vi "NewRobotTurningAroundBallDev.vi"(7 "firstCall?":bool, 8 "Target":dbl[](array[numeric]), 9 "KickToSkill in":refnum<class "KickToSkill.lvclass">, 10 "Game":refnum<class "Game.lvclass">, 11 "Robot in":refnum<class "Robot.lvclass">) -> (2 "KickToSkill out":refnum<class "KickToSkill.lvclass">, 3 "Robot out":refnum<class "Robot.lvclass">)   [LabVIEW 2021, in "KickToSkill.lvclass"]
uses:
  KickToSkill.lvclass
  Game_class/Game.lvclass
  Robot_class/Robot.lvclass
  robotTurningAroundBallStates.ctl
  Object_class/Object.lvclass/Object.ctl
  Game_class/Game.lvclass/Game.ctl
  Robot_class/Robot.lvclass/Robot.ctl
  <vilib>/Analysis/baseanly.llb/Unit Vector (DBL).vi
  <vilib>/Analysis/coordinate.llb/2D Cartesian Coordinate Rotation (Scalar).vi
  Robot_class/Read dest_x.vi
  Robot_class/Read dest_y.vi
  Robot_class/Read dest_orientation.vi
  Robot_class/Read kick_x.vi
  Robot_class/Read orientation.vi
  Game_class/Read BallRef.vi
  Object_class/Read position(x,y).vi
  Object_class/Read x.vi
  Robot_class/Write dest_orientation.vi
  Robot_class/Write dest_x.vi
  Robot_class/Write dest_y.vi
  Robot_class/Write kick_x.vi
  Robot_class/Write dribble.vi
  Ball_class/Ball.lvclass
  <vilib>/Analysis/NI_AALPro.lvlib
  <vilib>/Analysis/NI_AALBase.lvlib
panel:
  in  "Raio":dbl=200.0
  out "error out":errorcluster
  in  "error in (no error)":errorcluster
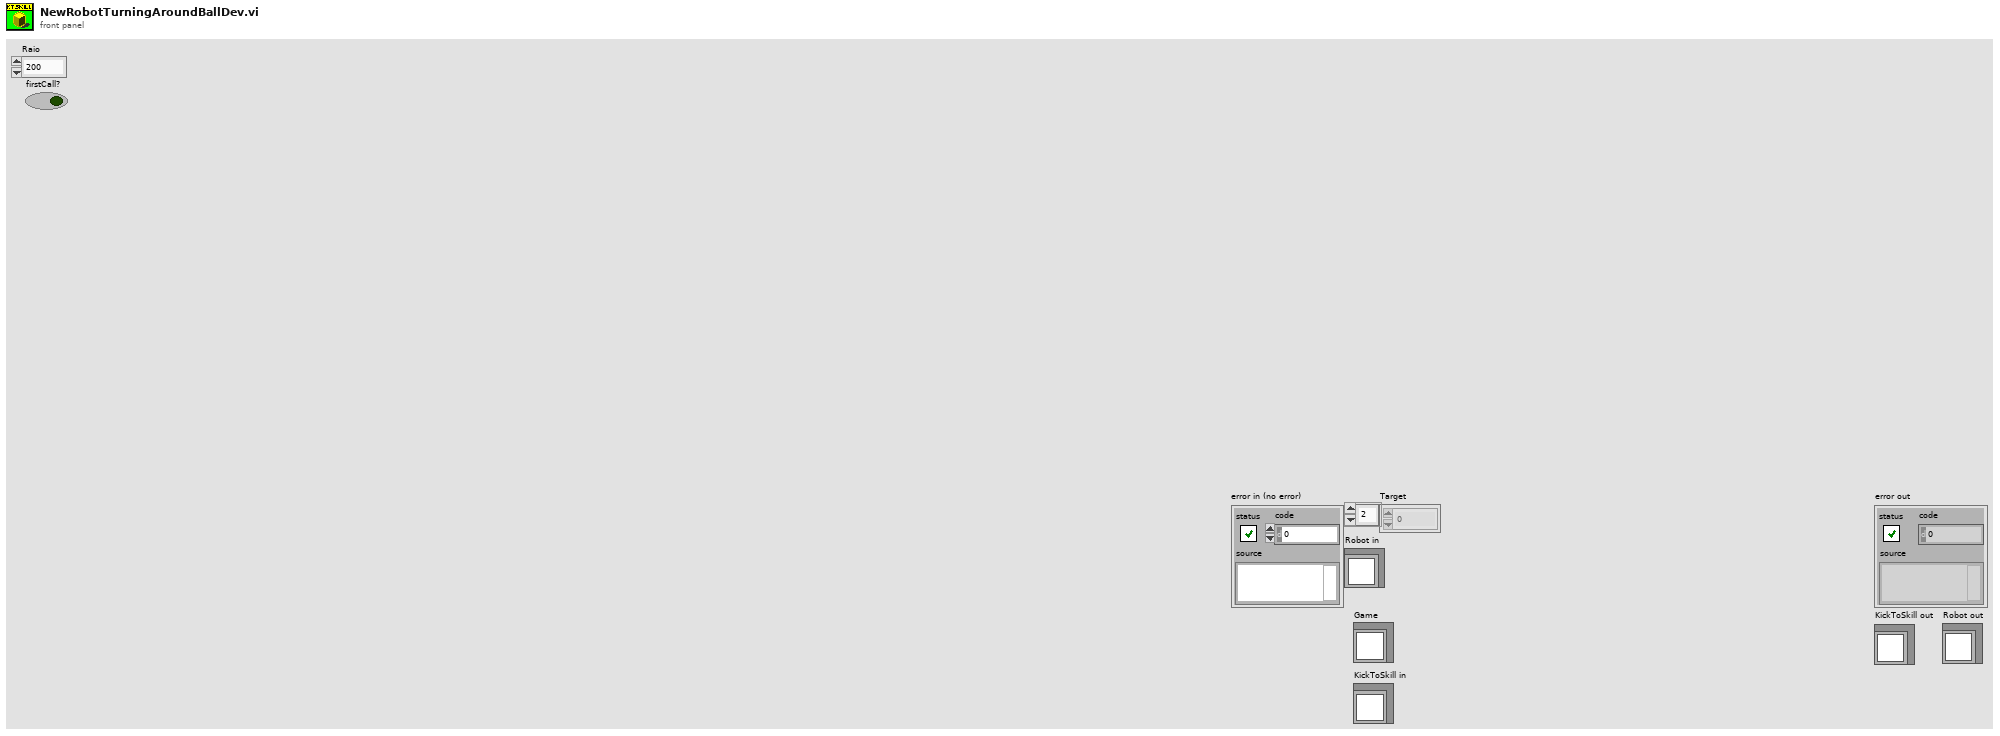
[diagram p1: front panel]
types:
  T1 = typedef "KickToSkill.lvclass/robotTurningAroundBallStates.ctl" = enum16{"go straight to the target", "go to point A", "circulating the ball", "take distance", "lining up", "shoot"}
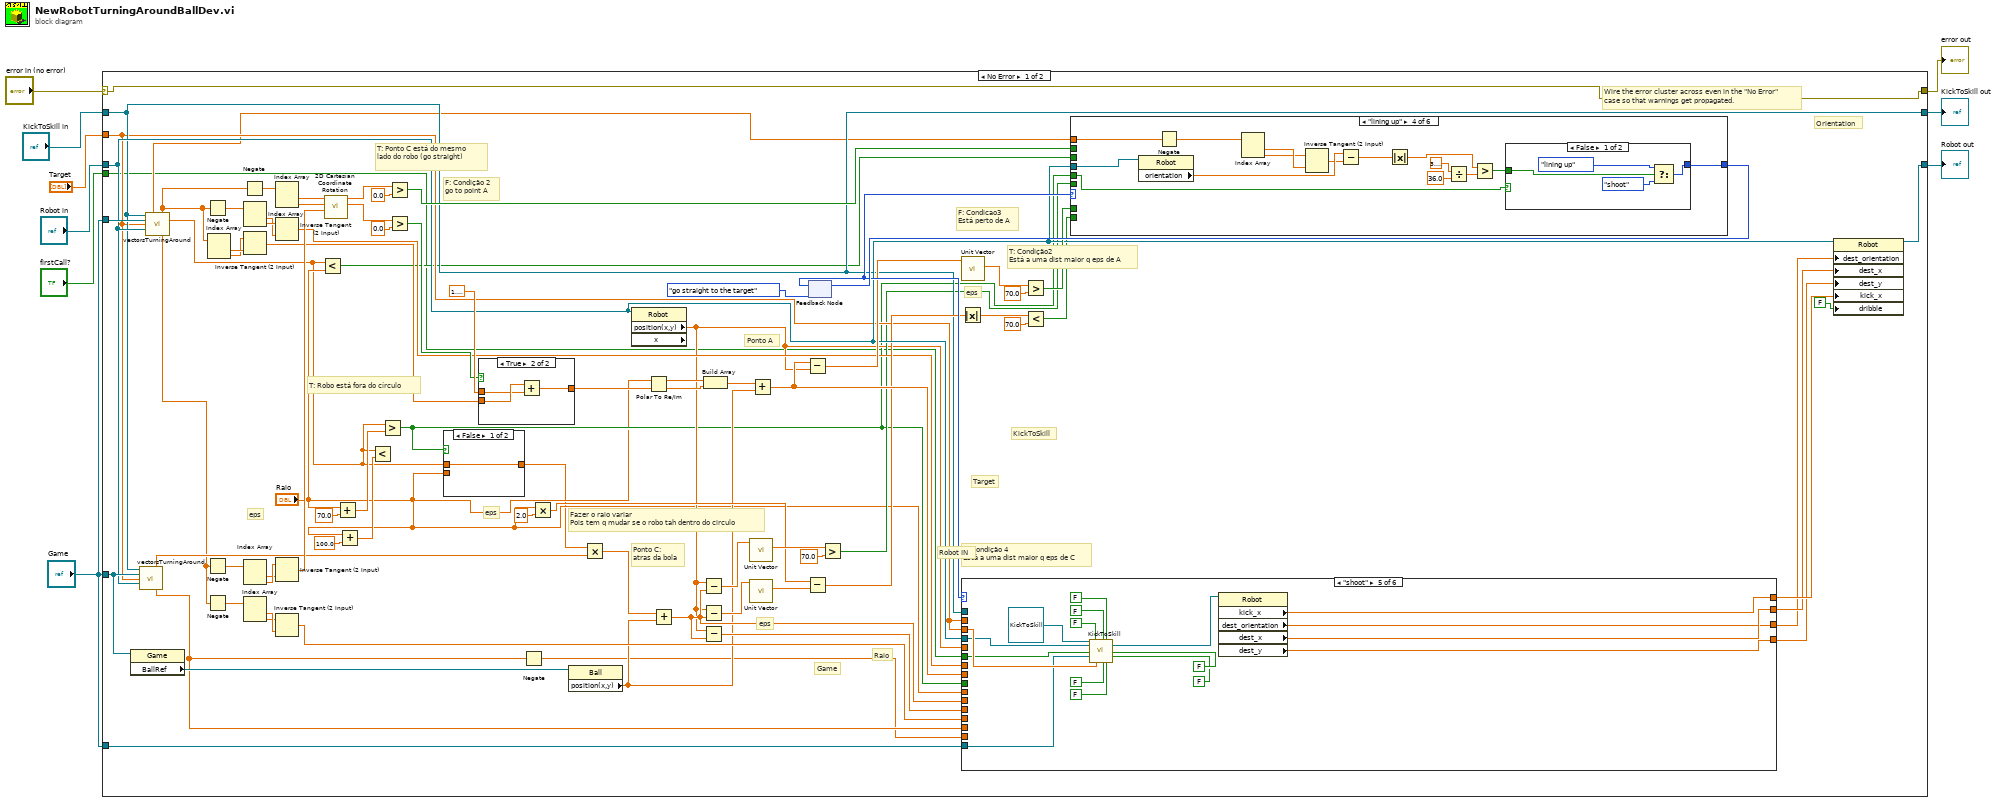
[diagram p0: block diagram]
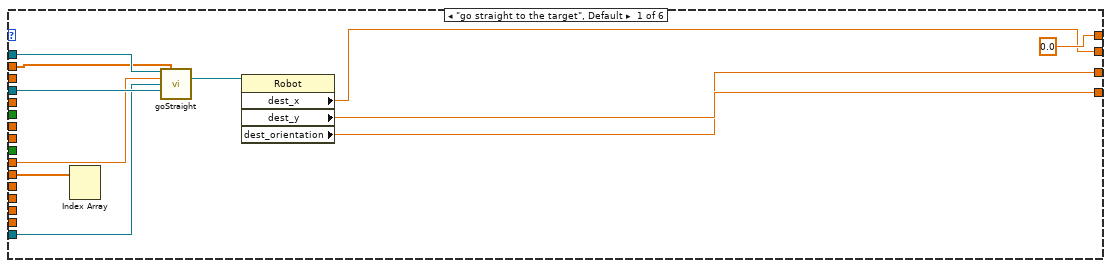
[diagram p3: hidden frame]
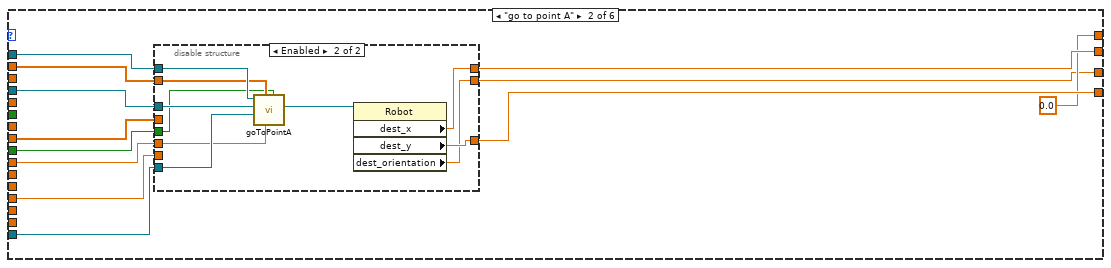
[diagram p4: hidden frame]
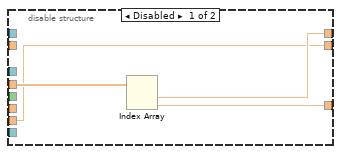
[diagram p5: hidden frame]
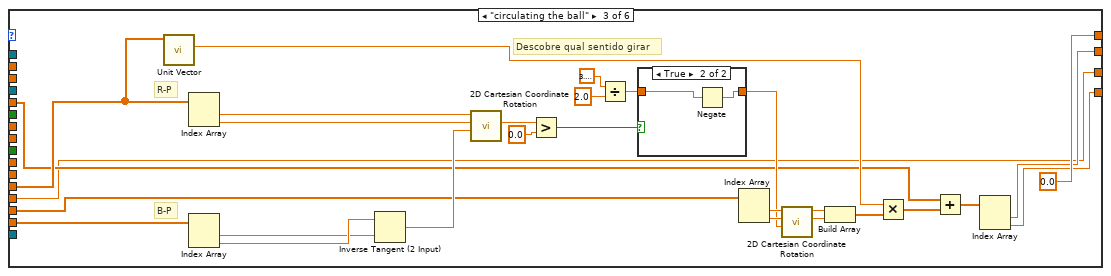
[diagram p6: hidden frame]
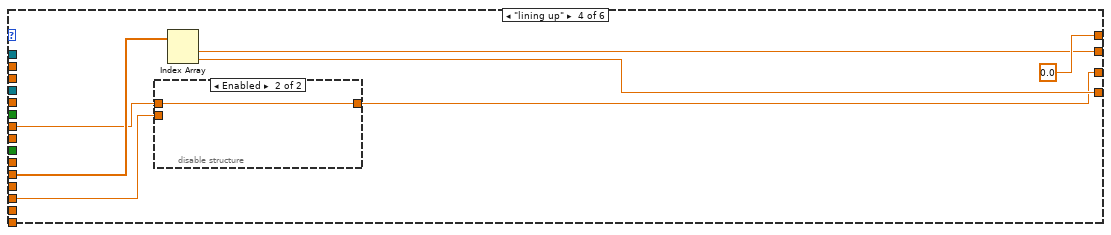
[diagram p8: hidden frame]
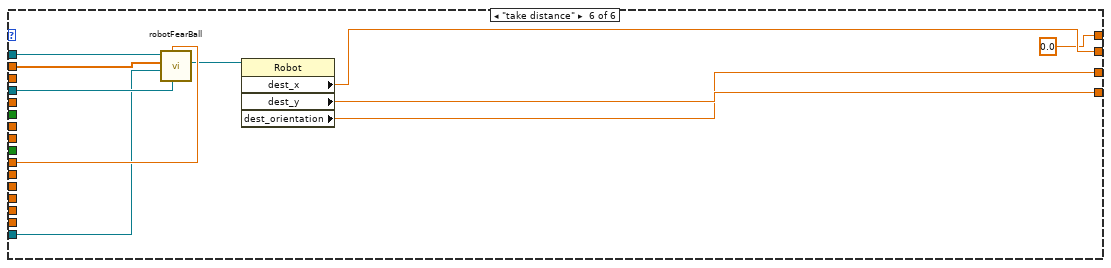
[diagram p10: hidden frame]
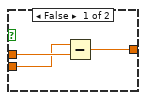
[diagram p11: hidden frame]
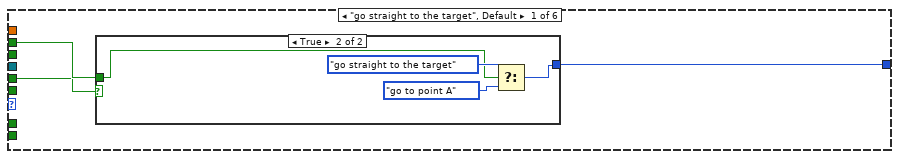
[diagram p12: hidden frame]
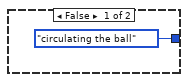
[diagram p13: hidden frame]
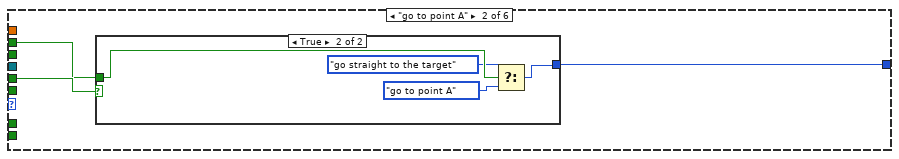
[diagram p14: hidden frame]
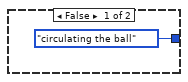
[diagram p15: hidden frame]
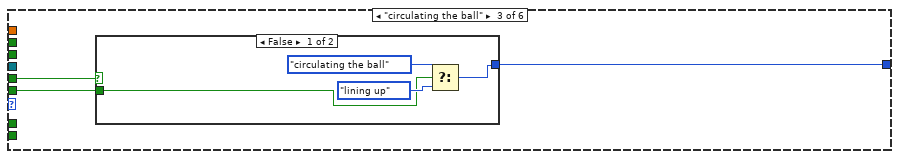
[diagram p16: hidden frame]
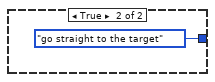
[diagram p17: hidden frame]
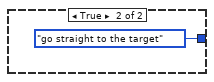
[diagram p18: hidden frame]
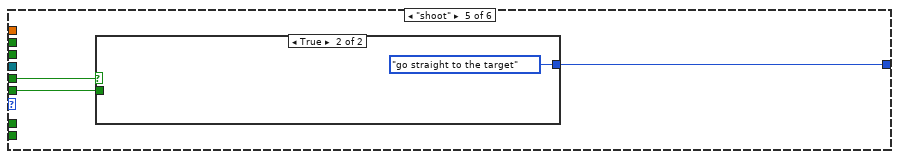
[diagram p19: hidden frame]
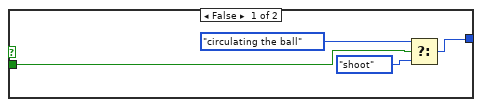
[diagram p20: hidden frame]
diagram:
  n1 = case shown="No Error" "error in (no error)" {
    selector: "error in (no error)" -> [w93 w268]
    tunnel: [w93 w268] -> w8
    tunnel: [w29 w267] -> w6
    tunnel: "KickToSkill in" -> [w29 w267]
    tunnel: "Robot in" -> [w45 w266]
    tunnel: [w92 w266] -> w4
    tunnel: "Target" -> [w28 _]
    tunnel: "Game" -> [w89 _]
    tunnel: "Game" -> [w46 _]
    tunnel: "Game" -> [w50 _]
    tunnel: "firstCall?" -> [w10 _]
    frame No Error {
      # "Fazer o raio variar\nPois tem q mudar se o robo tah dentro do circulo"
      # "Orientation"
      # "Raio"
      # "Robot IN"
      # "Game"
      # "KickToSkill"
      # "Target"
      # "eps"
      # "T: Condição 4\nEstá a uma dist maior q eps de C"
      # "F: Condicao3\nEstá perto de A"
      # "eps"
      # "Ponto C:\natras da bola"
      # "eps"
      # "eps"
      # "F: Condição 2\ngo to point A"
      # "T: Condição2\nEstá a uma dist maior q eps de A"
      # "Ponto A"
      # "T: Robo está fora do círculo"
      # "T: Ponto C está do mesmo lado do robo (go straight)"
      # "Wire the error cluster across even in the \"No Error\"\ncase so that warnings get propagated."
      n2 = property class="Game"(reference=w46) -> ("BallRef"=w68:refnum<class "Ball.lvclass">)  [unwired: 1 in, 2 out]
      n3 = call "vectorsTurningAround.vi"("KickToSkill in"=w29, "Game"=w46, "Target"=w28, "Robot in"=w45) -> ("B-T"=w69:dbl[], "R-B"=w31:dbl[])  [unwired: 4 in, 6 out]
      n4 = call "vectorsTurningAround.vi"("KickToSkill in"=w29, "Game"=w89, "Target"=w28, "Robot in"=w45) -> ("R-T"=w16:dbl[], "B-T"=w22:dbl[], "R-B norm"=w11:dbl, "R-B"=w34:dbl[])  [unwired: 4 in, 4 out]
      n5 = Negate(x=w22) -> (-x=w25:dbl[])
      n6 = Negate(x=w34) -> (-x=w33:dbl[])
      n7 = Negate(x=w34) -> (-x=w44:dbl[])
      n8 = Index Array(array=w22) -> (element #1=w80:dbl, element #2=w79:dbl)  [unwired: 2 in]
      n9 = Negate(x=w22) -> (-x=w78:dbl[])
      n10 = Index Array(array=w25) -> (element #1=w23:dbl, element #2=w24:dbl)  [unwired: 2 in]
      n11 = Inverse Tangent (2 Input)(1:w80, 2:w79) -> (0:w77:dbl)
      n12 = Index Array(array=w33) -> (element #1=w83:dbl, element #2=w84:dbl)  [unwired: 2 in]
      n13 = Index Array(array=w44) -> (element #1=w57:dbl, element #2=w56:dbl)  [unwired: 2 in]
      n14 = Index Array(array=w78) -> (element #1=w85:dbl, element #2=w86:dbl)  [unwired: 2 in]
      n15 = Inverse Tangent (2 Input)(1:w23, 2:w24) -> (0:w21:dbl)
      n16 = Inverse Tangent (2 Input)(1:w83, 2:w84) -> (0:w82:dbl)
      n17 = Inverse Tangent (2 Input)(1:w57, 2:w56) -> (0:w48:dbl)
      n18 = Less?(x=w11, y="Raio") -> (x < y?=w20:bool)
      n19 = call-poly <vilib>:"2D Cartesian Coordinate Rotation.vi"("theta"=w82, "y"=w86, "x"=w85) -> ("y out"=w75:dbl, "x out"=w87:dbl)  [unwired: 6 in, 1 out]
      n20 = Add(x="Raio", y=70.0) -> (x+y=w18:dbl)
      n21 = Add(x="Raio", y=100.0) -> (x+y=w26:dbl)
      n22 = Less?(x=w11, y=w26) -> ()  [unwired: 1 out]
      n23 = Greater?(x=w11, y=w18) -> (0:w14:bool)
      n24 = Greater?(x=w87, y=0.0) -> (0:w81:bool)
      n25 = Greater?(x=w75, y=0.0) -> (0:w73:bool)
      n26 = case shown="False" w14 {
        tunnel: "Raio" -> [_ w95]
        tunnel: [w94 w95] -> w12
        tunnel: w11 -> [w94 _]
        frame False {
        }
        frame True {
        }
      }
      n27 = case shown="True" w73 {
        tunnel: w77 -> [w201 w205]
        tunnel: 1.5707963267948966 -> [w202 w204]
        tunnel: [w200 w203] -> w63
        frame False {
          n28 = Subtract(x=w201, y=w202) -> (x-y=w200:dbl)
        }
        frame True {
          n29 = Add(x=w205, y=w204) -> (x+y=w203:dbl)
        }
      }
      n30 = Negate(x=w31) -> (-x=w30:dbl[])
      n31 = Multiply(x="Raio", y=2.0) -> (x*y=w39:dbl)
      n32 = property class="Ball"(reference=w68) -> ("position(x,y)"=w32:dbl[])  [unwired: 1 in, 2 out]
      n33 = Multiply(x=w12, y=w69) -> (x*y=w67:dbl[])
      n34 = property class="Robot" props=["position(x,y)", "x"](reference=w45) -> ("position(x,y)"=w15:dbl[])  [unwired: 1 in, 3 out]
      n35 = Polar To Re/Im(2:w63, 3:"Raio") -> (0:w61:dbl, 1:w62:dbl)
      n36 = Add(x=w67, y=w32) -> (x+y=w43:dbl[])
      n37 = Subtract(x=w15, y=w43) -> (x-y=w58:dbl[])
      n38 = Subtract(x=w15, y=w43) -> (x-y=w42:dbl[])
      n39 = Subtract(x=w15, y=w43) -> (x-y=w51:dbl[])
      n40 = Build Array(w62, w61) -> (w60:dbl[])
      n41 = call-poly <vilib>:"Unit Vector.vi"("Input Vector"=w58) -> ("norm"=w65:dbl)  [unwired: 8 in, 2 out]
      n42 = call-poly <vilib>:"Unit Vector.vi"("Input Vector"=w42) -> ("norm"=w41:dbl)  [unwired: 8 in, 2 out]
      n43 = Add(x=w60, y=w32) -> (x+y=w59:dbl[])
      n44 = Subtract(x=w59, y=w15) -> (x-y=w47:dbl[])
      n45 = Subtract(x=w39, y=w41) -> (x-y=w38:dbl)
      n46 = feedback #1(robotTurningAroundBallStates."go straight to the target") -> (w64:T1)
      n47 = Greater?(x=w65, y=70.0) -> (0:w17:bool)
      n48 = Absolute Value(x=w38) -> (abs(x)=w37:dbl)
      n49 = call-poly <vilib>:"Unit Vector.vi"("Input Vector"=w47) -> ("norm"=w71:dbl)  [unwired: 8 in, 2 out]
      n50 = case shown="\"shoot\"" w64 {
        tunnel: w59 -> [_ w118 _ _ _ _]
        tunnel: [0.0 ("kick_x") 0.0 ("kick_x") 0.0 ("kick_x") 0.0 ("kick_x") w173 0.0 ("kick_x")] -> w54
        tunnel: w43 -> [w105 _ _ w169 _ _]
        tunnel: [w99 w117 w135 w168 w177 w193] -> w53
        tunnel: [w98 w116 w134 w167 w176 w192] -> w52
        tunnel: w30 -> [_ _ w143 _ _ _]
        tunnel: w51 -> [_ _ w141 _ _ _]
        tunnel: w31 -> [_ _ w142 _ _ _]
        tunnel: w15 -> [_ _ w138 _ _ _]
        tunnel: w28 -> [_ _ _ _ w181 _]
        tunnel: w45 -> [w103 w114 _ _ w180 w196]
        tunnel: w50 -> [w96 w113 _ _ w179 w195]
        tunnel: w48 -> [_ w108 w133 w166 _ _]
        tunnel: [w97 w109 w133 w165 w175 w190] -> w49
        tunnel: w29 -> [w104 w115 _ _ _ w197]
        tunnel: "Raio" -> [w102 w112 _ _ _ w198]
        tunnel: w28 -> [w101 w111 _ _ _ w199]
        tunnel: w21 -> [_ _ _ w164 _ _]
        tunnel: w14 -> [_ w107 _ _ _ _]
        tunnel: w10 -> [_ _ _ _ w174 _]
        frame "go straight to the target", Default {
          n51 = Index Array(array=w105) -> ()  [unwired: 2 in, 2 out]
          n52 = call "goStraight.vi"("KickToSkill in"=w104, "Target"=w101, "Raio"=w102, "Game"=w96, "Robot in"=w103) -> ("Robot out"=w100:refnum<class "Robot.lvclass">)  [unwired: 8 in, 2 out]
          n53 = property class="Robot"(reference=w100) -> ("dest_x"=w99:dbl, "dest_y"=w98:dbl, "dest_orientation"=w97:dbl)  [unwired: 1 in, 2 out]
        }
        frame "go to point A" {
          n54 = disable-structure shown="Enabled" {
            disable-tunnel: w118 -> [w122 _]
            disable-tunnel: [w121 w126] -> w117
            disable-tunnel: [w120 w125] -> w116
            disable-tunnel: w115 -> [_ w132]
            disable-tunnel: w114 -> [_ w131]
            disable-tunnel: w113 -> [_ w130]
            disable-tunnel: w112 -> [_ w129]
            disable-tunnel: w111 -> [_ w128]
            disable-tunnel: [w119 w124] -> w109
            disable-tunnel: w108 -> [w119 _]
            disable-tunnel: w107 -> [_ w123]
            frame Disabled {
              n55 = Index Array(array=w122) -> (element #1=w121:dbl, element #2=w120:dbl)  [unwired: 2 in]
            }
            frame Enabled {
              n56 = call "goToPointA.vi"("Fora do circulo"=w123, "Raio"=w129, "Target"=w128, "Game"=w130, "Robot in"=w131, "KickToSkill in"=w132) -> ("Robot out"=w127:refnum<class "Robot.lvclass">)  [unwired: 3 in, 2 out]
              n57 = property class="Robot"(reference=w127) -> ("dest_x"=w126:dbl, "dest_y"=w125:dbl, "dest_orientation"=w124:dbl)  [unwired: 1 in, 2 out]
            }
          }
        }
        frame "circulating the ball" {
          # "B-P"
          # "R-P"
          # "Descobre qual sentido girar"
          n58 = call-poly <vilib>:"Unit Vector.vi"("Input Vector"=w141) -> ("norm"=w140:dbl)  [unwired: 8 in, 2 out]
          n59 = Index Array(array=w141) -> (element #1=w151:dbl, element #2=w150:dbl)  [unwired: 2 in]
          n60 = Index Array(array=w143) -> (element #1=w144:dbl, element #2=w145:dbl)  [unwired: 2 in]
          n61 = Inverse Tangent (2 Input)(1:w144, 2:w145) -> (0:w149:dbl)
          n62 = call-poly <vilib>:"2D Cartesian Coordinate Rotation.vi"("theta"=w149, "y"=w150, "x"=w151) -> ("y out"=w148:dbl)  [unwired: 6 in, 2 out]
          n63 = Greater?(x=w148, y=0.0) -> (0:w146:bool)
          n64 = Divide(x=3.141592653589793, y=2.0) -> (x/y=w153:dbl)
          n65 = case shown="True" w146 {
            tunnel: w153 -> [w161 w163]
            tunnel: [w161 w162] -> w152
            frame False {
            }
            frame True {
              n66 = Negate(x=w163) -> (-x=w162:dbl)
            }
          }
          n67 = Index Array(array=w142) -> (element #1=w159:dbl, element #2=w158:dbl)  [unwired: 2 in]
          n68 = call-poly <vilib>:"2D Cartesian Coordinate Rotation.vi"("theta"=w152, "y"=w158, "x"=w159) -> ("y out"=w156:dbl, "x out"=w157:dbl)  [unwired: 6 in, 1 out]
          n69 = Build Array(w157, w156) -> (w139:dbl[])
          n70 = Multiply(x=w140, y=w139) -> (x*y=w137:dbl[])
          n71 = Add(x=w138, y=w137) -> (x+y=w136:dbl[])
          n72 = Index Array(array=w136) -> (element #1=w135:dbl, element #2=w134:dbl)  [unwired: 2 in]
        }
        frame "lining up" {
          n73 = disable-structure shown="Enabled" {
            disable-tunnel: w166 -> [w171 _]
            disable-tunnel: [w171 w172] -> w165
            disable-tunnel: w164 -> [_ w172]
            frame Disabled {
            }
            frame Enabled {
            }
          }
          n74 = Index Array(array=w169) -> (element #1=w168:dbl, element #2=w167:dbl)  [unwired: 2 in]
        }
        frame "shoot" {
          n75 = call "KickToSkill.vi"("KickToSkill in"=refnum<class "KickToSkill.lvclass"> refnum, "Robot"=w180, "firstCall?"=w174, "Game"=w179, "use criteria?"=FALSE, "Target"=w181, "chipKick ?"=FALSE, "KickForce 0?"=FALSE, "WeakKick"=FALSE, "ForceInGame"=FALSE, "IgnorePosEst"=FALSE, "pass?"=FALSE) -> ("Robot out"=w183:refnum<class "Robot.lvclass">)  [unwired: 4 in, 3 out]
          n76 = property class="Robot"(reference=w183) -> ("kick_x"=w173:dbl, "dest_orientation"=w175:dbl, "dest_x"=w177:dbl, "dest_y"=w176:dbl)  [unwired: 1 in, 2 out]
        }
        frame "take distance" {
          n77 = call "robotFearBall.vi"("Robot in"=w196, "Raio"=w198, "Game"=w195, "Target"=w199, "KickToSkill in"=w197) -> ("Robot out"=w194:refnum<class "Robot.lvclass">)  [unwired: 4 in, 2 out]
          n78 = property class="Robot"(reference=w194) -> ("dest_x"=w193:dbl, "dest_y"=w192:dbl, "dest_orientation"=w190:dbl)  [unwired: 1 in, 2 out]
        }
      }
      n79 = Greater?(x=w71, y=70.0) -> (0:w70:bool)
      n80 = Less?(x=w37, y=70.0) -> (x < y?=w35:bool)
      n81 = case shown="\"lining up\"" w64 {
        tunnel: [w208 w216 w224 w231 w252 w259] -> w91
        tunnel: w81 -> [w207 w214 _ _ _ w260]
        tunnel: w14 -> [w206 w215 w223 w230 w250 _]
        tunnel: w70 -> [_ _ _ _ _ _]
        tunnel: w45 -> [_ _ _ w244 _ _]
        tunnel: w35 -> [_ _ _ _ _ _]
        tunnel: w16 -> [_ _ _ w236 _ _]
        tunnel: w20 -> [_ _ _ _ _ w258]
        tunnel: w17 -> [_ _ w222 _ w251 _]
        frame "go straight to the target", Default {
          n82 = case shown="True" w206 {
            tunnel: [robotTurningAroundBallStates."circulating the ball" w212] -> w208
            tunnel: w207 -> [_ w210]
            frame False {
            }
            frame True {
              n83 = Select(t=robotTurningAroundBallStates."go straight to the target", s=w210, f=robotTurningAroundBallStates."go to point A") -> (s? t:f=w212:T1)
            }
          }
        }
        frame "go to point A" {
          n84 = case shown="True" w215 {
            tunnel: [robotTurningAroundBallStates."circulating the ball" w218] -> w216
            tunnel: w214 -> [_ w221]
            frame False {
            }
            frame True {
              n85 = Select(t=robotTurningAroundBallStates."go straight to the target", s=w221, f=robotTurningAroundBallStates."go to point A") -> (s? t:f=w218:T1)
            }
          }
        }
        frame "circulating the ball" {
          n86 = case shown="False" w223 {
            tunnel: [w227 robotTurningAroundBallStates."go straight to the target"] -> w224
            tunnel: w222 -> [w225 _]
            frame False {
              n87 = Select(t=robotTurningAroundBallStates."circulating the ball", s=w225, f=robotTurningAroundBallStates."lining up") -> (s? t:f=w227:T1)
            }
            frame True {
            }
          }
        }
        frame "lining up" {
          n88 = property class="Robot"(reference=w244) -> ("orientation"=w243:dbl)  [unwired: 1 in, 2 out]
          n89 = Negate(x=w236) -> (-x=w235:dbl[])
          n90 = Index Array(array=w235) -> (element #1=w234:dbl, element #2=w233:dbl)  [unwired: 2 in]
          n91 = Inverse Tangent (2 Input)(1:w234, 2:w233) -> (0:w232:dbl)
          n92 = Subtract(x=w243, y=w232) -> (x-y=w242:dbl)
          n93 = Absolute Value(x=w242) -> (abs(x)=w241:dbl)
          n94 = Divide(x=3.141592653589793, y=36.0) -> (x/y=w238:dbl)
          n95 = Greater?(x=w241, y=w238) -> (0:w237:bool)
          n96 = case shown="False" w230 {
            tunnel: w237 -> [w248 _]
            tunnel: [w245 robotTurningAroundBallStates."go straight to the target"] -> w231
            frame False {
              n97 = Select(t=robotTurningAroundBallStates."lining up", s=w248, f=robotTurningAroundBallStates."shoot") -> (s? t:f=w245:T1)
            }
            frame True {
            }
          }
        }
        frame "shoot" {
          n98 = case shown="True" w250 {
            tunnel: [w255 robotTurningAroundBallStates."go straight to the target"] -> w252
            tunnel: w251 -> [w253 _]
            frame False {
              n99 = Select(t=robotTurningAroundBallStates."circulating the ball", s=w253, f=robotTurningAroundBallStates."shoot") -> (s? t:f=w255:T1)
            }
            frame True {
            }
          }
        }
        frame "take distance" {
          n100 = case shown="False" w260 {
            tunnel: [w262 robotTurningAroundBallStates."go straight to the target"] -> w259
            tunnel: w258 -> [w261 _]
            frame False {
              n101 = Select(t=robotTurningAroundBallStates."take distance", s=w261, f=robotTurningAroundBallStates."circulating the ball") -> (s? t:f=w262:T1)
            }
            frame True {
            }
          }
        }
      }
      n102 = feedback-in #1(w91) -> ()
      n103 = property class="Robot"(reference=w45, "dest_orientation"=w49, "dest_x"=w53, "dest_y"=w52, "kick_x"=w54, "dribble"=FALSE) -> (reference out=w92:refnum<class "Robot.lvclass">)  [unwired: 1 in, 1 out]
    }
    frame Error {
    }
  }
  "error out" <- w8
  "KickToSkill out" <- w6
  "Robot out" <- w4
